vi "Cleanup.vi"(8 "error in (no error)":errorcluster, 11 "Effect in":refnum<class "Effect.lvclass">) -> (0 "error out":errorcluster)   [LabVIEW 2018, in "Effect.lvclass"]
uses:
  Effect.lvclass
  Effect.lvclass/Effect.ctl
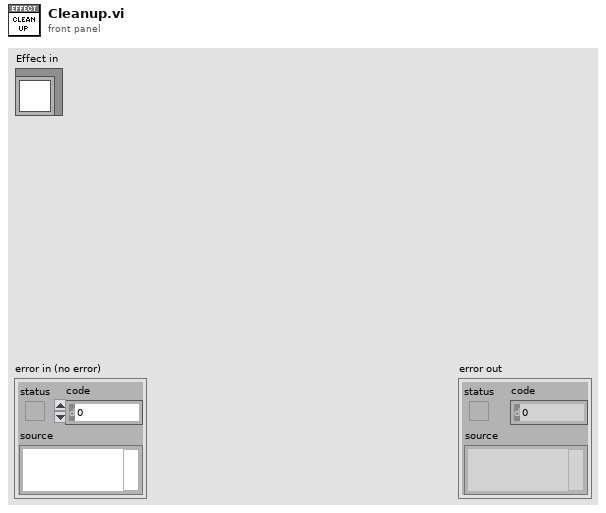
[diagram p1: front panel]
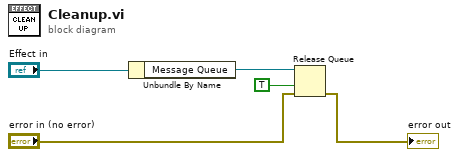
[diagram p0: block diagram]
diagram:
  n1 = Unbundle By Name("Effect in") -> ("Message Queue"=w2:refnum<queue>)
  n2 = Release Queue(queue=w2, force destroy? (F)=TRUE, error in (no error)="error in (no error)") -> (error out=→"error out":errorcluster)  [unwired: 2 out]
